vi "GetChannelData.vi"(0 "SmartScope in":refnum<k24>, 1 "LatestDataPackage":refnum<k24>, 2 "AnalogChannel":refnum<k24>) -> (3 "SmartScope out":refnum<k24>, 4 "Waveform Graph":dbl[](array[numeric]), 5 "ViewportBegin":dbl, 6 "ViewportEnd":dbl)   [LabVIEW 2015]
uses:
  C:/LabNation/SmartScopeApp/SmartScope/bin/Windows/AnyCPU/Debug/LabNation.DeviceInterface.dll
  LabNation/SmartScopeApp/SmartScope/bin/Windows/AnyCPU/Debug/LabNation.DeviceInterface.dll
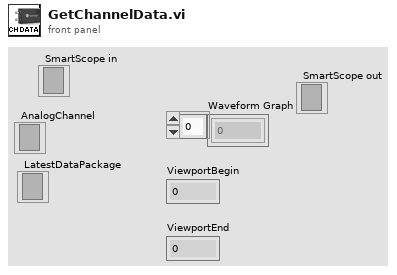
[diagram p1: front panel]
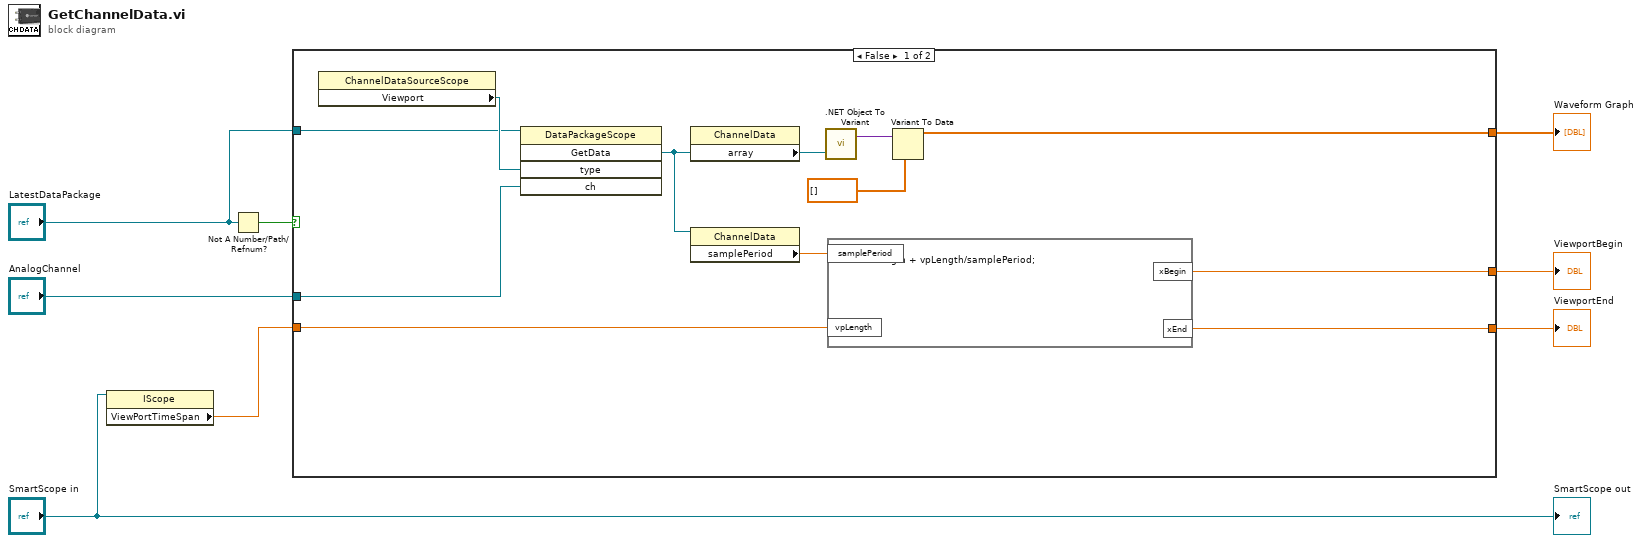
[diagram p0: block diagram]
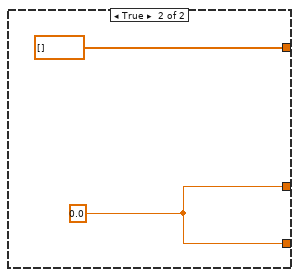
[diagram p2: hidden frame]
diagram:
  n1 = property class="IScope"(reference="SmartScope in") -> ("ViewPortTimeSpan"=w1:dbl)  [unwired: 1 in, 2 out]
  n2 = Not A Number/Path/Refnum?(number/path/refnum="LatestDataPackage") -> (NaN/Path/Refnum?=w7:bool)
  n3 = case shown="False" w7 {
    tunnel: "LatestDataPackage" -> [w15 _]
    tunnel: w1 -> [w13 _]
    tunnel: [w12 dbl[] [] ("Waveform Graph")] -> w6
    tunnel: [w11 w21] -> w4
    tunnel: [w10 w21] -> w5
    tunnel: "AnalogChannel" -> [w9 _]
    frame False {
      n4 = property class="ChannelDataSourceScope"() -> ("Viewport"=w20:refnum<k24>)  [unwired: 2 in, 2 out]
      n5 = invoke class="DataPackageScope" method="GetData"(reference=w15, "type"=w20, "ch"=w9) -> ("GetData"=w16:refnum<k24>)  [unwired: 2 in, 4 out]
      n6 = property class="ChannelData"(reference=w16) -> ("array"=w19:refnum<k24>)  [unwired: 1 in, 2 out]
      n7 = property class="ChannelData"(reference=w16) -> ("samplePeriod"=w14:dbl)  [unwired: 1 in, 2 out]
      n8 = call <vilib>:".NET Object To Variant.vi"(".NET object"=w19) -> ("variant"=w17:variant)  [unwired: 1 in, 1 out]
      n9 = formula code="xBegin = 0;\nxEnd = xBegin + vpLength/samplePeriod;"("samplePeriod"=w14, "vpLength"=w13) -> ("xBegin"=w11:dbl, "xEnd"=w10:dbl)
      n10 = Variant To Data(type=dbl[] [] ("Waveform Graph"), Variant=w17) -> (data=w12:dbl[])  [unwired: 1 in, 1 out]
    }
    frame True {
      w21 = 0.0 ("xBegin")
    }
  }
  "Waveform Graph" <- w6
  "ViewportEnd" <- w5
  "ViewportBegin" <- w4
  "SmartScope out" <- "SmartScope in"
